vi "close arduino.vi"(8 "error in (no error)":errorcluster, 11 "Arduino Resource Out":T1) -> (0 "error out":errorcluster)   [LabVIEW 2016]
uses:
  <vilib>/LabVIEW Interface for Arduino/Type Defs/Arduino Resource.ctl
  <vilib>/LabVIEW Interface for Arduino/Type Defs/Board Type.ctl
  <vilib>/LabVIEW Interface for Arduino/LabVIEW Interface for Arduino.lvlib
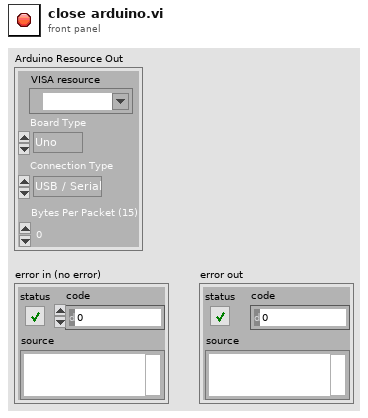
[diagram p1: front panel]
types:
  T1 = typedef "LabVIEW Interface for Arduino.lvlib/Arduino Resource.ctl" = cluster{"VISA resource":refnum<visa-resource-name>, "Board Type":T2, "Connection Type":enum8{"USB / Serial"}, "Bytes Per Packet (15)":u8}
  T2 = typedef "LabVIEW Interface for Arduino.lvlib/Board Type.ctl" = enum16{"Uno", "Dimuelanove w/Atmega 328", "Mega 2560"}
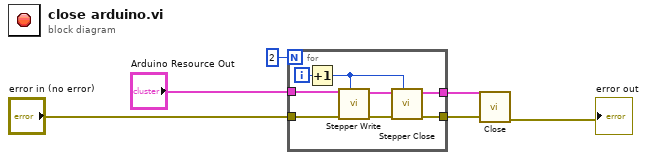
[diagram p0: block diagram]
diagram:
  n1 = for {
    N: 2 -> [_]
    tunnel: [w14] -> w6
    tunnel: "Arduino Resource Out" -> [w11]
    tunnel: "error in (no error)" -> [w8]
    tunnel: [w7] -> w5
    i -> [w13]
    n2 = Increment(x=w13) -> (x+1=w9:i32)
    n3 = call <vilib>:"Stepper Write.vi"("Stepper #"=w9, "error in"=w8, "Arduino Resource"=w11) -> ("error out"=w12:errorcluster, "Arduino Resource Out"=w10:T1)  [unwired: 7 in]
    n4 = call <vilib>:"Stepper Close.vi"("Stepper #"=w9, "error in"=w12, "Arduino Resource"=w10) -> ("error out"=w7:errorcluster, "Arduino Resource Out"=w14:T1)  [unwired: 7 in]
  }
  n5 = call <vilib>:"Close.vi"("Arduino Resource"=w6, "error in"=w5) -> ("error out"=→"error out":errorcluster)  [unwired: 13 in]
